vi "Teardown UE Loop.vi"(11 "ABD Panel in":refnum<class "ABD Panel.lvclass">) -> (0 "error out":errorcluster)   [LabVIEW 2021, in "ABD Panel.lvclass"]
uses:
  ABD Panel.lvclass
  ABD Panel.lvclass/ABD Panel.ctl
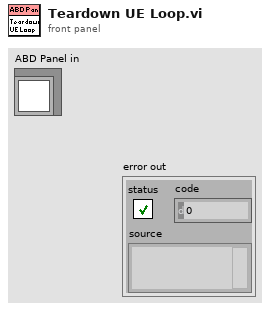
[diagram p1: front panel]
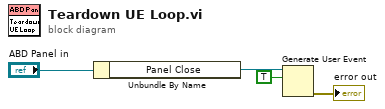
[diagram p0: block diagram]
diagram:
  n1 = Unbundle By Name("ABD Panel in") -> ("Panel Close"=w2:refnum<user-event>)
  n2 = Generate User Event(user event=w2, event data cluster=TRUE ("event data")) -> (error out=→"error out":errorcluster)  [unwired: 2 in, 1 out]
